vi "prueba DAQ.vi"() -> ()   [LabVIEW 2010]
panel:
  in  "DAQ Controls":T1={"Minimum Value"=-10.0, "Maximum Value"=10.0, "Physical Channel"="Dev1/ao0", "DAQ Fs (S/s)"=10000.0} {"Minimum Value" min=-10.0 max=0.0; "Maximum Value" min=0.0 max=10.0}
  out "En Funcionamiento?":bool
  in  "Calibracion DAQ":T2
  out "Waveform":waveform(dbl)(graph)
  in  "tiempo (ms)":dbl
  in  "DAQ?":bool
  in  "stop":bool
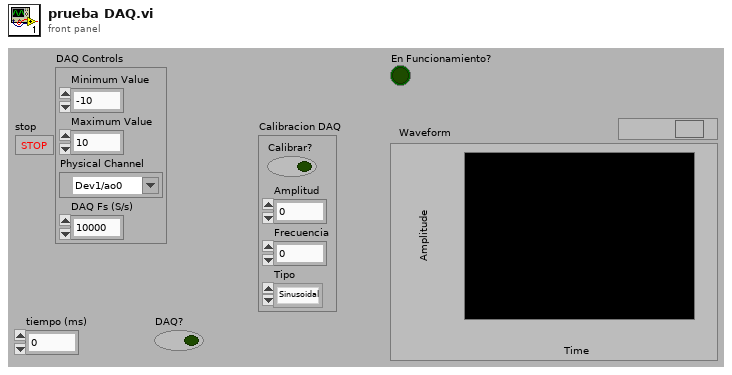
[diagram p1: front panel]
types:
  T1 = cluster{"Minimum Value":dbl, "Maximum Value":dbl, "Physical Channel":tag, "DAQ Fs (S/s)":dbl}
  T2 = cluster{"Calibrar?":bool, "Amplitud":dbl, "Frecuencia":dbl, "Tipo":enum16{"Sinusoidal", "Triangular", "Cuadrada"}}
  T3 = cluster{"DAQ Fs (S/s)":dbl, "task":refnum<k21>, "error":errorcluster, "Min Value":dbl, "Max Value":dbl}
  T4 = cluster{"DAQ Limits":cluster{"max":dbl, "min":dbl}, "Control Limits":cluster{"max":dbl, "min":dbl}}
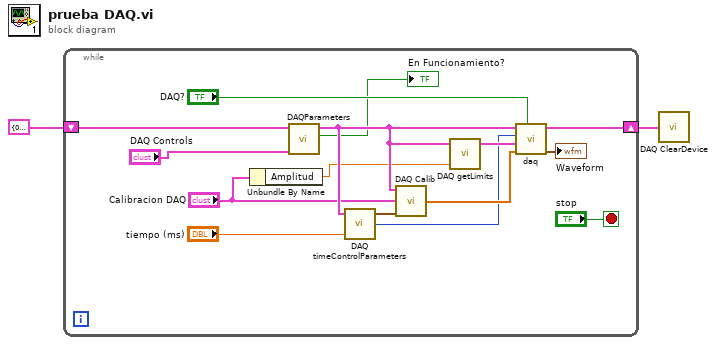
[diagram p0: block diagram]
diagram:
  n1 = while {
    shift-right: [w16] -> w1
    shift-left: T3 {"DAQ Fs (S/s)"=0.0, "task"="", "error"={"status"=TRUE, "code"=0, "source"=""}, "Min Value"=0.0, "Max Value"=0.0} ("DAQ Device OUT") -> [w13]
    stop <- "stop" stop-if-true
    n2 = Unbundle By Name("Calibracion DAQ") -> ("Amplitud"=w6:dbl)
    n3 = call "DAQParameters.vi"("DAQ Controls"="DAQ Controls", "DAQ Device IN"=w13) -> ("En Funcionamiento?"=→"En Funcionamiento?":bool, "DAQ Device OUT"=w10:T3)  [unwired: 4 in]
    n4 = call "DAQ timeControlParameters.vi"("tiempo (ms)"="tiempo (ms)", "DAQ Device IN"=w10) -> ("#samples"=w9:u32, "Time Control Parameters"=w11:cluster{"# samples":u32, "tiempos (ms)":dbl})  [unwired: 2 in]
    n5 = call "DAQ Calib.vi"("Time Control Parameters"=w11, "Calibracion DAQ"="Calibracion DAQ", "DAQ Device IN"=w10) -> ("Calibration OUT"=w15:dbl[])  [unwired: 1 in]
    n6 = call "DAQ getLimits.vi"("Amplitud"=w6, "DAQ Device IN"=w10) -> ("Limites"=w14:T4)  [unwired: 3 in]
    n7 = call "daq.vi"("DAQ?"="DAQ?", "Control Array"=w15, "Limites"=w14, "#samples"=w9, "DAQ Device IN"=w10) -> ("Waveform Graph"=→"Waveform":waveform(dbl), "DAQ Device OUT"=w16:T3)  [unwired: 2 in]
  }
  n8 = call "DAQ ClearDevice.vi"("DAQ Device IN"=w1) -> ()
